vi "Init VCG50.vi"(8 "error in (no error)":errorcluster, 11 "VGC50 In":T1={"serial settings"={"port"="", "baud rate"=115200}, "device information"={"type"="", "model number"="", "serial number"="", "firmware version"="", "hardware version"=""}, "VGC"=refnum, "Backing SP"={"mode"=0, "thresholds"={"lower"=0.0, "upper"=0.0}, "on"=FALSE}, "Chamber SP"={"mode"=1, "thresholds"={"lower"=0.0, "upper"=0.0}, "on"=FALSE}} {"Chamber SP"."thresholds"."upper" format="%#_5p"; "Chamber SP"."thresholds"."lower" format="%#_5p"; "Chamber SP"."mode" items=["off", "on", "channel 1", "channel 2", "channel 3"]; "Backing SP"."thresholds"."upper" format="%#_5p"; "Backing SP"."thresholds"."lower" format="%#_5p"; "Backing SP"."mode" items=["off", "on", "channel 1", "channel 2", "channel 3"]; "serial settings"."baud rate" items=["9600"=9600, "19200"=19200, "38400"=38400, "57600"=57600, "115200"=115200]}) -> (0 "error out":errorcluster, 3 "VGC50 Out":T1={"serial settings"={"port"="", "baud rate"=115200}, "device information"={"type"="", "model number"="", "serial number"="", "firmware version"="", "hardware version"=""}, "VGC"=refnum, "Backing SP"={"mode"=0, "thresholds"={"lower"=0.0, "upper"=0.0}, "on"=FALSE}, "Chamber SP"={"mode"=1, "thresholds"={"lower"=0.0, "upper"=0.0}, "on"=FALSE}} {"Chamber SP"."thresholds"."upper" format="%#_5p"; "Chamber SP"."thresholds"."lower" format="%#_5p"; "Chamber SP"."mode" items=["off", "on", "channel 1", "channel 2", "channel 3"]; "Backing SP"."thresholds"."upper" format="%#_5p"; "Backing SP"."thresholds"."lower" format="%#_5p"; "Backing SP"."mode" items=["off", "on", "channel 1", "channel 2", "channel 3"]; "serial settings"."baud rate" items=["9600"=9600, "19200"=19200, "38400"=38400, "57600"=57600, "115200"=115200]})   [LabVIEW 2024]
uses:
  controls/VGC50.ctl
  <instrlib>/PL Inficon VGC/PL Inficon VGC.lvclass
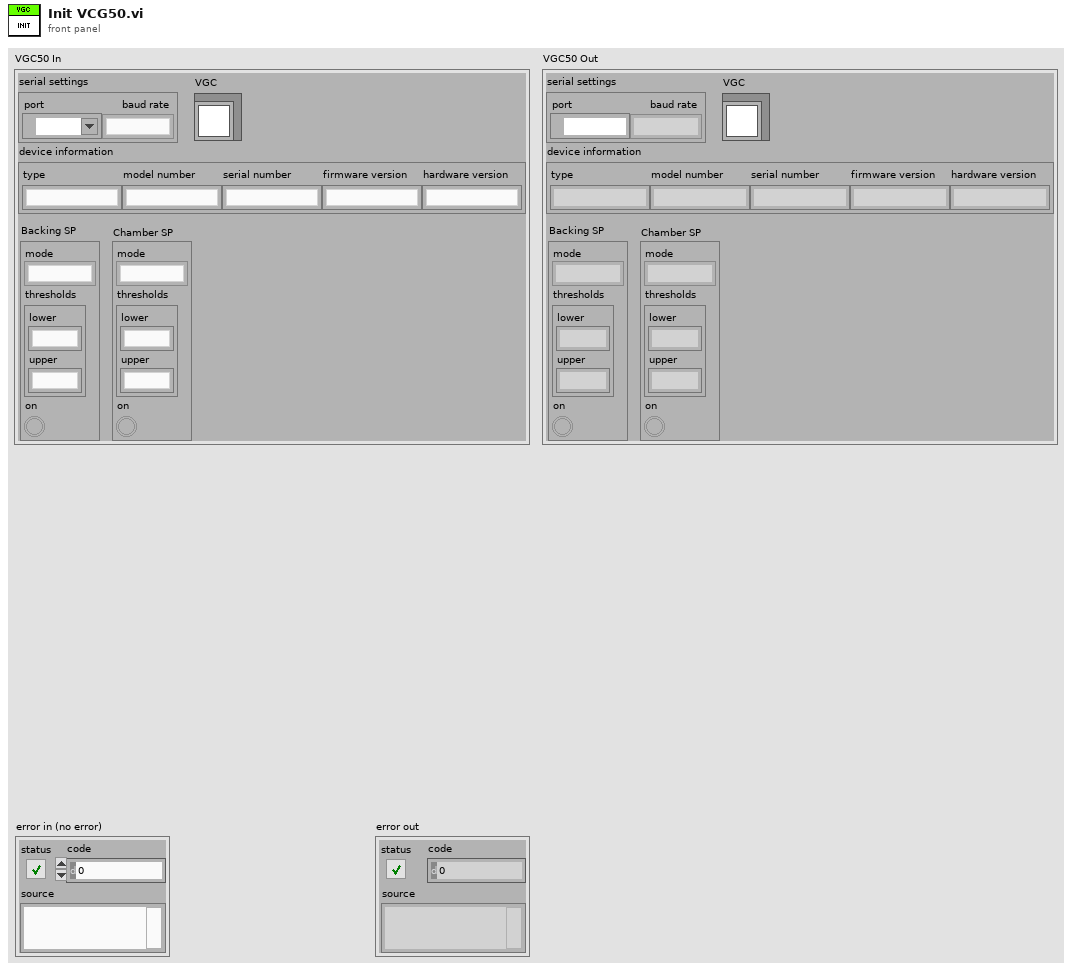
[diagram p1: front panel]
types:
  T1 = typedef "VGC50.ctl" = cluster{"serial settings":cluster{"port":refnum<visa-resource-name>, "baud rate":u32}, "device information":cluster{"type":string, "model number":string, "serial number":string, "firmware version":string, "hardware version":string}, "VGC":refnum<class "PL Inficon VGC.lvclass">, "Backing SP":cluster{"mode":u16, "thresholds":cluster{"lower":dbl, "upper":dbl}, "on":bool}, "Chamber SP":cluster{"mode":u16, "thresholds":cluster{"lower":dbl, "upper":dbl}, "on":bool}}
  T2 = cluster{"type":string, "model number":string, "serial number":string, "firmware version":string, "hardware version":string}
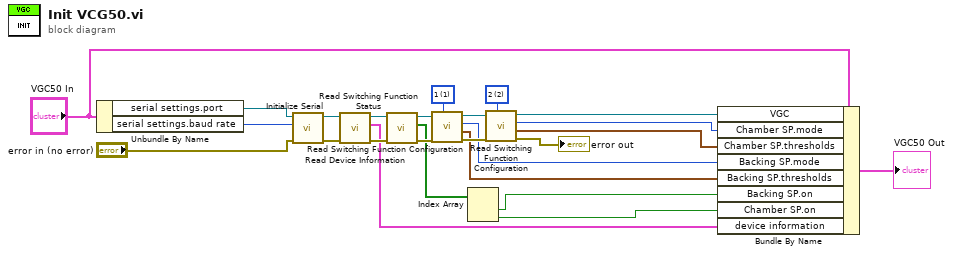
[diagram p0: block diagram]
diagram:
  w12 = u16 2 items=["1"=1, "2"=2, "3"=3, "4"=4, "5"=5, "6"=6] ("function")
  w13 = u16 1 items=["1"=1, "2"=2, "3"=3, "4"=4, "5"=5, "6"=6] ("function")
  n1 = Unbundle By Name("VGC50 In") -> ("serial settings.port"=w25:refnum<visa-resource-name>, "serial settings.baud rate"=w24:u32)
  n2 = call <instrlib>:"Initialize Serial.vi"("error in (no error)"="error in (no error)", "baud rate (115200)"=w24, "port"=w25) -> ("error out"=w21:errorcluster, "VGC out"=w22:refnum<class "PL Inficon VGC.lvclass">)  [unwired: 7 in]
  n3 = call <instrlib>:"Read Device Information.vi"("error in (no error)"=w21, "VGC in"=w22) -> ("error out"=w18:errorcluster, "information"=w2:T2, "VGC out"=w19:refnum<class "PL Inficon VGC.lvclass">)  [unwired: 7 in]
  n4 = call <instrlib>:"Read Switching Function Status.vi"("error in (no error)"=w18, "VGC in"=w19) -> ("error out"=w16:errorcluster, "status"=w5:bool[], "VGC out"=w17:refnum<class "PL Inficon VGC.lvclass">)  [unwired: 7 in]
  n5 = call <instrlib>:"Read Switching Function Configuration.vi"("function"=w13, "error in (no error)"=w16, "VGC in"=w17) -> ("error out"=w14:errorcluster, "thresholds"=w6:cluster{"lower":dbl, "upper":dbl}, "mode"=w7:u16, "VGC out"=w15:refnum<class "PL Inficon VGC.lvclass">)  [unwired: 5 in]
  n6 = Index Array(array=w5) -> (element #1=w4:bool, element #2=w3:bool)  [unwired: 2 in]
  n7 = call <instrlib>:"Read Switching Function Configuration.vi"("function"=w12, "error in (no error)"=w14, "VGC in"=w15) -> ("error out"=→"error out":errorcluster, "thresholds"=w8:cluster{"lower":dbl, "upper":dbl}, "mode"=w9:u16, "VGC out"=w10:refnum<class "PL Inficon VGC.lvclass">)  [unwired: 5 in]
  n8 = Bundle By Name(cluster="VGC50 In", "VGC"=w10, "Chamber SP.mode"=w9, "Chamber SP.thresholds"=w8, "Backing SP.mode"=w7, "Backing SP.thresholds"=w6, "Backing SP.on"=w4, "Chamber SP.on"=w3, "device information"=w2) -> (→"VGC50 Out":T1)
